vi "Configure Loopback Value.vi"(7 "Use Counter?":bool, 8 "error in (no error)":errorcluster, 9 "Value":u8, 10 "FPGA VI Reference in":refnum<k20>, 11 "SLSC EDS System Tests in":refnum<class "SLSC EDS System Tests.lvclass">) -> (0 "error out":errorcluster, 2 "FPGA VI Reference Out":refnum<k20>, 3 "SLSC EDS System Tests out":refnum<class "SLSC EDS System Tests.lvclass">)   [LabVIEW 2015, in "SLSC EDS System Tests.lvclass"]
uses:
  SLSC EDS System Tests.lvclass
  <vilib>/Utility/error.llb/Error Cluster From Error Code.vi
  <vilib>/rvi/errors/niLvFpgaAdjustHostInterfaceError.vi
  <vilib>/rvi/interface/nirviReadWriteControl/nirviReadWriteControl.xnode
  NiFpgaLv.dll
  <vilib>/rvi/interface/Simulation/niFpgaSimulationCallBeginRW.vi
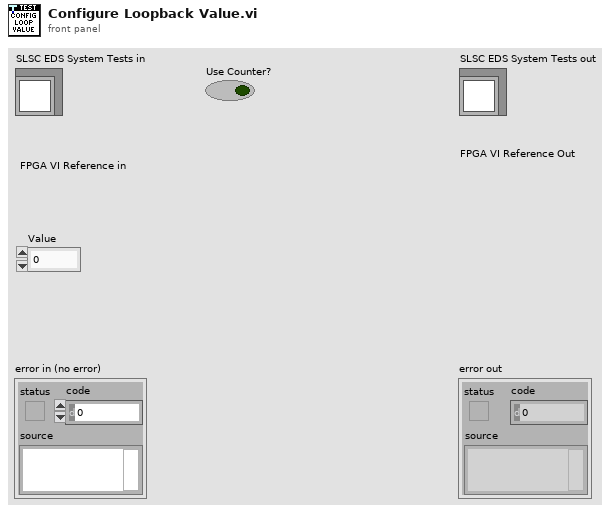
[diagram p1: front panel]
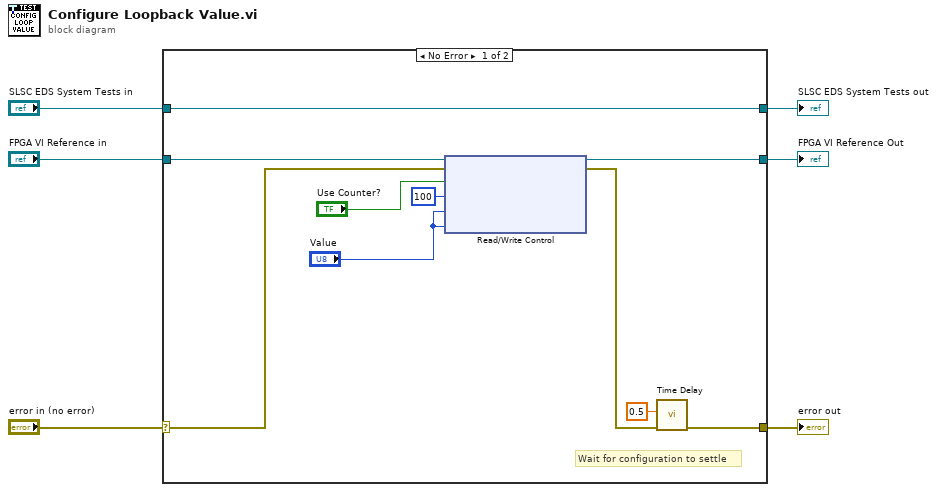
[diagram p0: block diagram]
diagram:
  n1 = case shown="No Error" "error in (no error)" {
    selector: "error in (no error)" -> [w14 w19]
    tunnel: [w8 w19] -> w5
    tunnel: [w16 w18] -> w3
    tunnel: "SLSC EDS System Tests in" -> [w16 w18]
    tunnel: "FPGA VI Reference in" -> [w15 w17]
    tunnel: [w13 w17] -> w1
    frame No Error {
      # "Wait for configuration to settle"
      n2 = xnode "Read/Write Control"("FPGA VI Reference In"=w15, "error in"=w14, "Use Counter?"="Use Counter?", "Wait (mSec)"=u32 100, "Connector0/DIOPORT3"="Value", "Connector0/DIOPORT0"="Value") -> ("FPGA VI Reference Out"=w13:refnum<k20>, "error out"=w9:errorcluster)
      n3 = call "Time Delay"("error in (no error)"=w9, "Delay Time (s)"=0.5) -> ("error out"=w8:errorcluster)  [unwired: 9 in]
    }
    frame Error {
    }
  }
  "error out" <- w5
  "SLSC EDS System Tests out" <- w3
  "FPGA VI Reference Out" <- w1
